vi "AccessConfigCluster.vi"() -> ()   [LabVIEW 2012]
uses:
  Config.ctl
  ConfigKey.ctl
  C:/ConfigKeyTypes.ctl
panel:
  in  "ConfigKey":T1
  in  "Numeric":i32=5000
  in  "Action":enum16{"Read", "Write"}(ring)
  in  "Input":T3={"variant"=variant, "Type"=enum."Int"}
  out "Value 2":string
  out "Class Name":string
  out "Value":string
  out "Found?":bool
  in  "ControlName":string
  in  "Config":T4
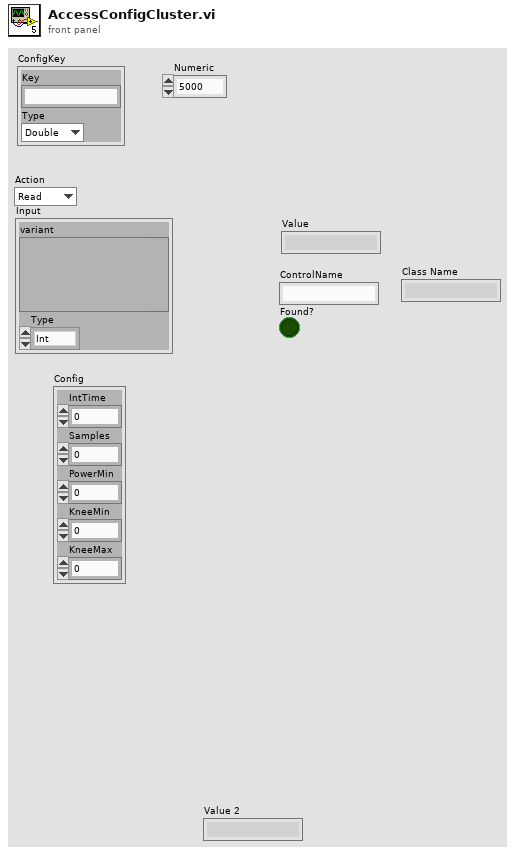
[diagram p1: front panel]
types:
  T1 = typedef "ConfigKey.ctl" = cluster{"Key":string, "Type":T2}
  T2 = typedef "ConfigKeyTypes.ctl" = enum16{"Double", "Int", "String"}
  T3 = cluster{"variant":variant, "Type":enum16{"Double", "Int", "String"}}
  T4 = typedef "Config.ctl" = cluster{"IntTime":i32, "Samples":i32, "PowerMin":dbl, "KneeMin":dbl, "KneeMax":dbl}
  T5 = cluster{"Variant":variant, "Type":enum16{"Double", "Int", "String"}}
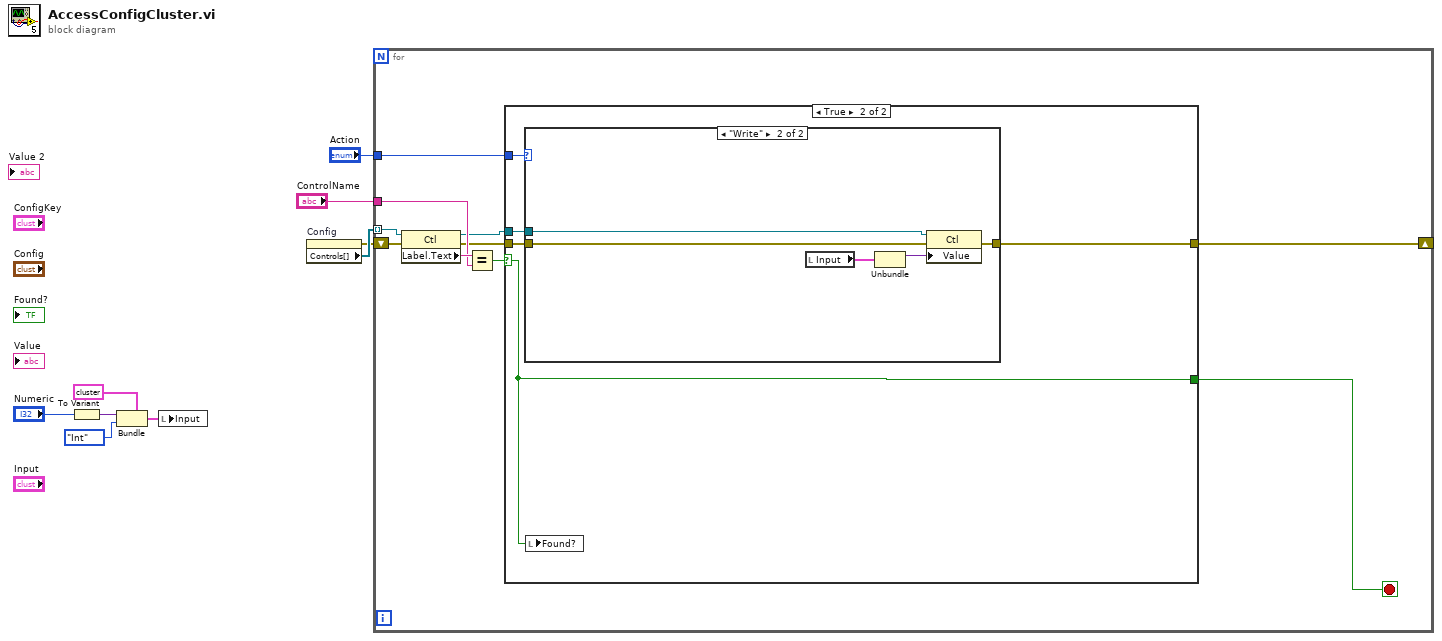
[diagram p0: block diagram]
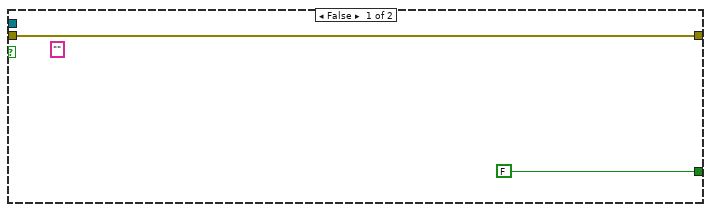
[diagram p2: hidden frame]
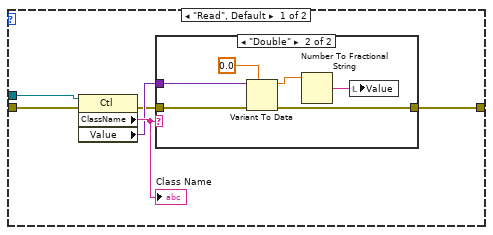
[diagram p3: hidden frame]
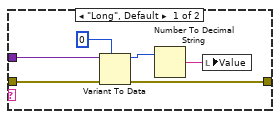
[diagram p4: hidden frame]
diagram:
  n1 = To Variant(anything="Numeric") -> (Variant=w5:variant)
  n2 = Bundle(cluster=T5 {"Variant"=variant, "Type"=enum."Double"}, "Variant"=w5, "Type"=enum16{"Double", "Int", "String"}."Int") -> (w2:T5)
  n3 = local write "Input"(w2) -> ()
  n4 = property on="Config" class="Clust (strict)"() -> (error out=w8:errorcluster, "Controls[]"=w9:refnum<vi>[])  [unwired: 2 in, 1 out]
  n5 = for {
    tunnel: w9 -> [w19] mode=indexing
    tunnel: "ControlName" -> [w16]
    shift-right: [w13] -> _
    shift-left: w8 -> [w18]
    tunnel: "Action" -> [w11]
    stop <- w12 stop-if-true
    n6 = property class="Ctl"(reference=w19, error in=w18) -> (reference out=w10:refnum<vi>, error out=w14:errorcluster, "Label.Text"=w17:string)
    n7 = Equal?(x=w17, y=w16) -> (x = y?=w15:bool)
    n8 = case shown="True" w15 {
      selector: w15 -> [_ w26]
      tunnel: w14 -> [w21 w24]
      tunnel: [w21 w22] -> w13
      tunnel: [FALSE w26] -> w12
      tunnel: w11 -> [_ w25]
      tunnel: w10 -> [_ w23]
      frame False {
        (unwired) ""
      }
      frame True {
        n9 = case shown="\"Write\"" w25 {
          tunnel: w24 -> [w31 w47]
          tunnel: w23 -> [w28 w46]
          tunnel: [w27 w45] -> w22
          frame "Read", Default {
            n10 = property class="Ctl"(reference=w28, error in=w31) -> (error out=w29:errorcluster, "ClassName"=w32:string, "Value"=w30:variant)  [unwired: 1 out]
            "Class Name" <- w32
            n11 = case shown="\"Double\"" w32 {
              tunnel: w30 -> [w38 w43]
              tunnel: w29 -> [w36 w42]
              tunnel: [w35 w41] -> w27
              frame "Long", Default {
                n12 = Variant To Data(error in=w36, type=0, Variant=w38) -> (data=w34:i32, error out=w35:errorcluster)
                n13 = Number To Decimal String(number=w34) -> (decimal integer string=w33:string)  [unwired: 1 in]
                n14 = local write "Value"(w33) -> ()
              }
              frame "Double" {
                n15 = Variant To Data(error in=w42, type=0.0, Variant=w43) -> (data=w40:dbl, error out=w41:errorcluster)
                n16 = Number To Fractional String(number=w40) -> (F-format string=w39:string)  [unwired: 3 in]
                n17 = local write "Value"(w39) -> ()
              }
            }
          }
          frame "Write" {
            n18 = local read "Input"() -> (w49:T3)
            n19 = Unbundle(w49) -> ("variant"=w48:variant)  [unwired: 1 out]
            n20 = property class="Ctl"(reference=w46, error in=w47, "Value"=w48) -> (error out=w45:errorcluster)  [unwired: 1 out]
          }
        }
        n21 = local write "Found?"(w26) -> ()
      }
    }
  }
